vi "Is Nominal State.vi"(11 "Base Event in":refnum<class "Base Event.lvclass">) -> (2 "Is Nominal State?":bool)   [LabVIEW 2021, in "jettl.lvlib" / "Base Event.lvlib" / "Base Event.lvclass"]
uses:
  Base Event.lvclass
  Base Event.lvclass/Base Event.ctl
  State/Nominal State/Nominal State.lvclass
  C:/git/jettl/jettl/jettl/Base Event/State/Nominal State/Nominal State.lvclass
  C:/git/jettl/jettl/jettl/Base Event/State/State/State.lvclass
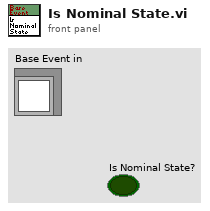
[diagram p1: front panel]
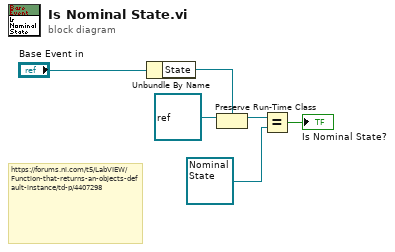
[diagram p0: block diagram]
diagram:
  # "https://forums.ni.com/t5/LabVIEW/Function-that-returns-an-objects-default-instance/td-p/4407298"
  n1 = Unbundle By Name("Base Event in") -> ("State"=w4:refnum<class "State.lvclass">)
  n2 = Preserve Run-Time Class(object in=refnum<class> refnum ("LabVIEW Object"), 2:w4) -> (object out=w5:refnum<class "State.lvclass">)  [unwired: 1 in, 1 out]
  n3 = Equal?(x=w5, y=refnum<class "Nominal State.lvclass"> refnum ("jettl.lvlib:Base Event.lvlib:State.lvlib:Nominal State.lvclass")) -> (x = y?=→"Is Nominal State?":bool)
